vi "CreaInformeExcel.vi"(0 "UnidadesF":refnum<vi>, 1 "ValorParoDesplazamiento":dbl, 2 "TipusAssaig":string, 3 "ActivaParoDefor":bool, 4 "VelocidadEnsayo":dbl, 5 "ArraiMostresxProva":dbl[](array[numeric]), 6 "Nom Assaig":string, 7 "Precarga":bool, 8 "NºTests":u8, 9 "ValorPrecarga":dbl, 10 "UnidadesD":refnum<vi>, 11 "ActivaParoRotura":bool, 12 "TablaFinal":dbl[][](array[numeric]), 13 "ValorParoRotura":dbl) -> (14 "status":bool)   [LabVIEW 2017]
uses:
  <vilib>/addons/_office/excel.llb/Excel Easy Table (num).vi
  <vilib>/addons/_office/excel.llb/Excel Easy Table (str).vi
  <vilib>/Utility/NIReport.llb/NI_report.lvclass
  <vilib>/addons/_office/NI_ReportGenerationToolkit.lvlib
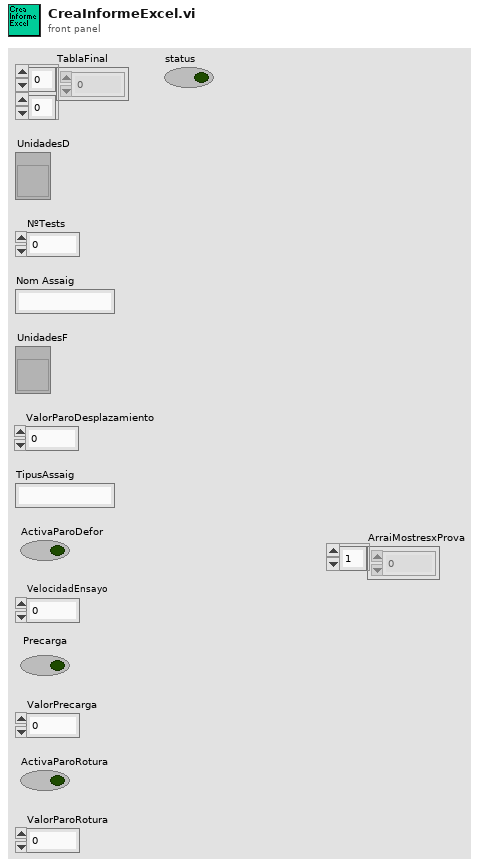
[diagram p1: front panel]
types:
  T1 = enum16{"maximized", "minimized", "normal", "no change"}
  T2 = enum16{"Standard Report", "HTML", "Word", "Excel"}
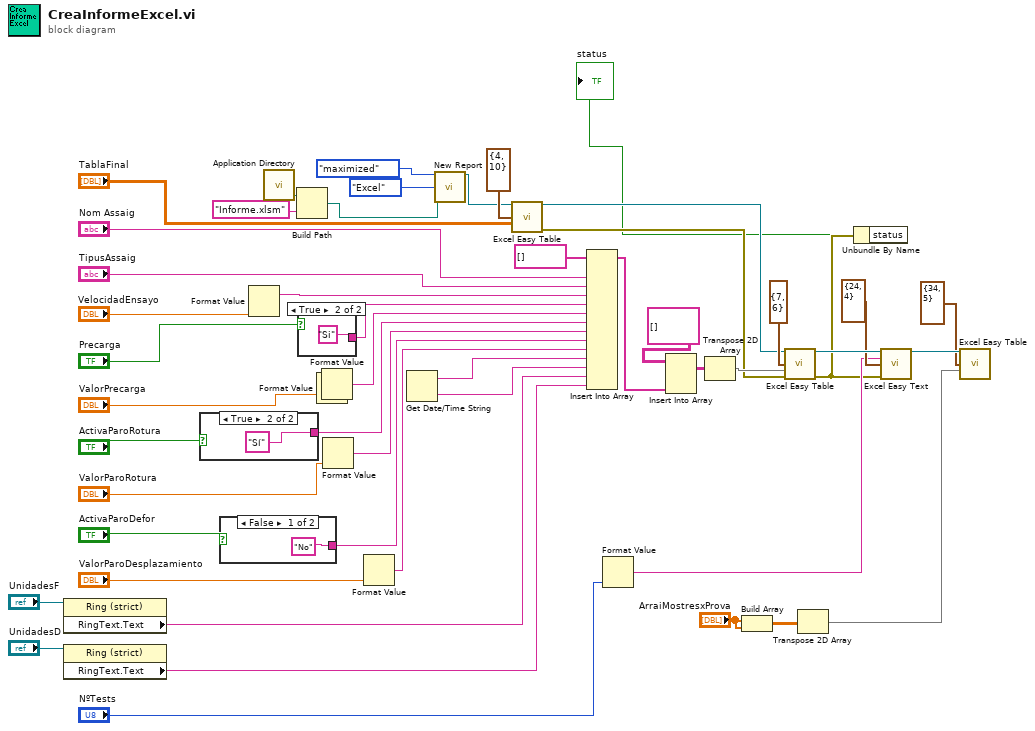
[diagram p0: block diagram]
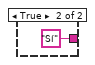
[diagram p2: hidden frame]
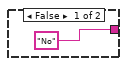
[diagram p3: hidden frame]
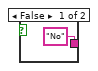
[diagram p4: hidden frame]
diagram:
  n1 = property on="Property Node" class="Ring (strict)"(reference="UnidadesF") -> ("RingText.Text"=w8:string)  [unwired: 1 in, 2 out]
  n2 = property on="Property Node" class="Ring (strict)"(reference="UnidadesD") -> ("RingText.Text"=w9:string)  [unwired: 1 in, 2 out]
  n3 = case shown="True" "ActivaParoRotura" {
    tunnel: ["No" "Sí"] -> w38
    frame False {
    }
    frame True {
    }
  }
  n4 = case shown="False" "ActivaParoDefor" {
    tunnel: ["No" "Sí"] -> w40
    frame False {
    }
    frame True {
    }
  }
  n5 = Format Value(value (0)="VelocidadEnsayo") -> (output string=w30:string)  [unwired: 2 in]
  n6 = call <vilib>:"Application Directory.vi"() -> ("Application Directory"=w16:path)
  n7 = Build Path(base path=w16, name or relative path="Informe.xlsm") -> (appended path=w18:path)
  n8 = case shown="True" "Precarga" {
    tunnel: ["No" "Si"] -> w35
    frame False {
    }
    frame True {
    }
  }
  n9 = Format Value() -> ()  [unwired: 3 in, 1 out]
  n10 = Format Value(value (0)="ValorPrecarga") -> (output string=w37:string)  [unwired: 2 in]
  n11 = Format Value(value (0)="ValorParoRotura") -> (output string=w39:string)  [unwired: 2 in]
  n12 = Format Value(value (0)="ValorParoDesplazamiento") -> (output string=w41:string)  [unwired: 2 in]
  n13 = Get Date/Time String() -> (date string=w7:string, time string=w6:string)  [unwired: 3 in]
  n14 = call <vilib>:"New Report.vi"("window state (normal)"=T1."maximized", "report type"=T2."Excel", "template (empty)"=w18) -> ("report out"=w20:refnum<class "NI_report.lvclass">)  [unwired: 11 in, 1 out]
  n15 = call-poly <vilib>:"Excel Easy Table.vi"("report in"=w20, "start (0, 0)"=cluster{"row":i32, "column":i32} {"row"=4, "column"=10}, "text data"="TablaFinal") -> ("report out"=w25:refnum<class "NI_report.lvclass">, "error out"=w26:errorcluster)  [unwired: 8 in, 3 out]
  n16 = Insert Into Array(array=string[] [] ("new element/subarray"), new element #1="Nom Assaig", new element #2="TipusAssaig", new element #3=w30, new element #4=w35, new element #5=w37, new element #6=w38, new element #7=w39, new element #8=w40, new element #9=w41, new element #10=w7, new element #11=w6, new element #12=w8, new element #13=w9) -> (w32:string[])  [unwired: 1 in]
  n17 = Format Value(value (0)="NºTests") -> (output string=w46:string)  [unwired: 2 in]
  n18 = Insert Into Array(array=string[][] [] ("text data"), new element=w32) -> (w34:string[][])  [unwired: 2 in]
  n19 = Transpose 2D Array(2D array=w34) -> (transposed array=w33:string[][])
  n20 = Build Array("ArraiMostresxProva", "ArraiMostresxProva") -> (w2:dbl[][])
  n21 = call-poly <vilib>:"Excel Easy Table.vi"("report in"=w25, "start (0, 0)"=cluster{"row":i32, "column":i32} {"row"=7, "column"=6}, "text data"=w33, "error in (no error)"=w26) -> ("report out"=w48:refnum<class "NI_report.lvclass">, "error out"=w44:errorcluster)  [unwired: 7 in, 3 out]
  n22 = Transpose 2D Array(2D array=w2) -> (transposed array=w1:dbl[][])
  n23 = Unbundle By Name(w44) -> ("status"=→"status":bool)
  n24 = call <vilib>:"Excel Easy Text.vi"("report in"=w48, "text"=w46, "start (-1, -1)"=cluster{"row":i32, "column":i32} {"row"=24, "column"=4} ("start (0, 0)"), "error in (no error)"=w44) -> ("report out"=w5:refnum<class "NI_report.lvclass">)  [unwired: 7 in, 4 out]
  n25 = call-poly <vilib>:"Excel Easy Table.vi"("report in"=w5, "start (0, 0)"=cluster{"row":i32, "column":i32} {"row"=34, "column"=5}, "text data"=w1) -> ()  [unwired: 8 in, 5 out]
